vi "AutoaimVar.vi"() -> ()   [LabVIEW 2016]
panel:
  in  "jostle":bool
  out "Light in Use":bool
  out "Blink the Light":bool
  in  "reverse":bool
  out "Left Joystick Value":dbl
  out "Winch Run Speed":dbl
  in  "Winch Fast Run":bool
  in  "Drive First Run":bool
  out "Session Target":dbl
  out "Session Center":dbl
  in  "Target Acquired":bool
  in  "Panic Reached":bool
  in  "Winch Panic":bool
  in  "Autoaim New Session":bool
  in  "Autoaim Epsilon":bool
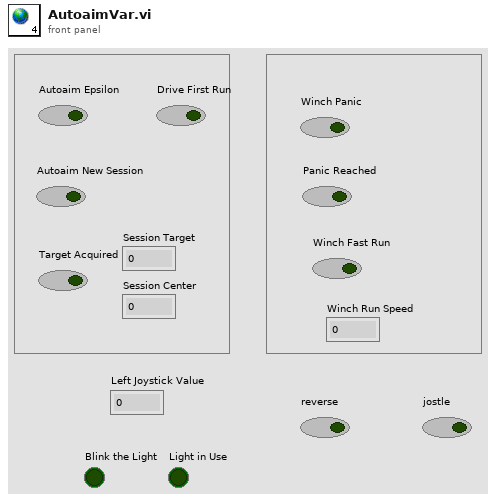
[diagram p1: front panel]
diagram:
